vi "Example Solver.vi"(10 "Word List":string[](array[string])=["YELLOW", "ORANGE", "PURPLE", "BLUE", "GREEN", "RED"], 11 "Word Search Grid":string[][](array[string])=[["R", "B", "L", "U", "E", "W"], ["E", "G", "N", "A", "R", "O"], ["D", "B", "C", "E", "W", "L"], ["L", "L", "D", "K", "V", "L"], ["P", "U", "R", "P", "L", "E"], ["N", "E", "E", "R", "G", "Y"]]) -> (3 "Solutions":T1={"BLUE"=[{"Row"=0, "Column"=1}, {"Row"=0, "Column"=2}, {"Row"=0, "Column"=3}, {"Row"=0, "Column"=4}], "GREEN"=[{"Row"=5, "Column"=4}, {"Row"=5, "Column"=3}, {"Row"=5, "Column"=2}, {"Row"=5, "Column"=1}, {"Row"=5, "Column"=0}], "ORANGE"=[{"Row"=1, "Column"=5}, {"Row"=1, "Column"=4}, {"Row"=1, "Column"=3}, {"Row"=1, "Column"=2}, {"Row"=1, "Column"=1}, {"Row"=1, "Column"=0}], "PURPLE"=[{"Row"=4, "Column"=0}, {"Row"=4, "Column"=1}, {"Row"=4, "Column"=2}, {"Row"=4, "Column"=3}, {"Row"=4, "Column"=4}, {"Row"=4, "Column"=5}], "RED"=[{"Row"=0, "Column"=0}, {"Row"=1, "Column"=0}, {"Row"=2, "Column"=0}], "YELLOW"=[{"Row"=5, "Column"=5}, {"Row"=4, "Column"=5}, {"Row"=3, "Column"=5}, {"Row"=2, "Column"=5}, {"Row"=1, "Column"=5}, {"Row"=0, "Column"=5}]})   [LabVIEW 2023]
uses:
  Solutions--map.ctl
  Letter Index--cluster.ctl
panel:
  # "Do not change the connector pane of this VI."
  # "Observe the default values stored in this VI to understand how each word is represented in the Solutions map.\n\nSee the block diagram for a simple implementation of a solution. Note that this approach is not very efficient, and you will want to come up with a faster way to find the words in the grid."
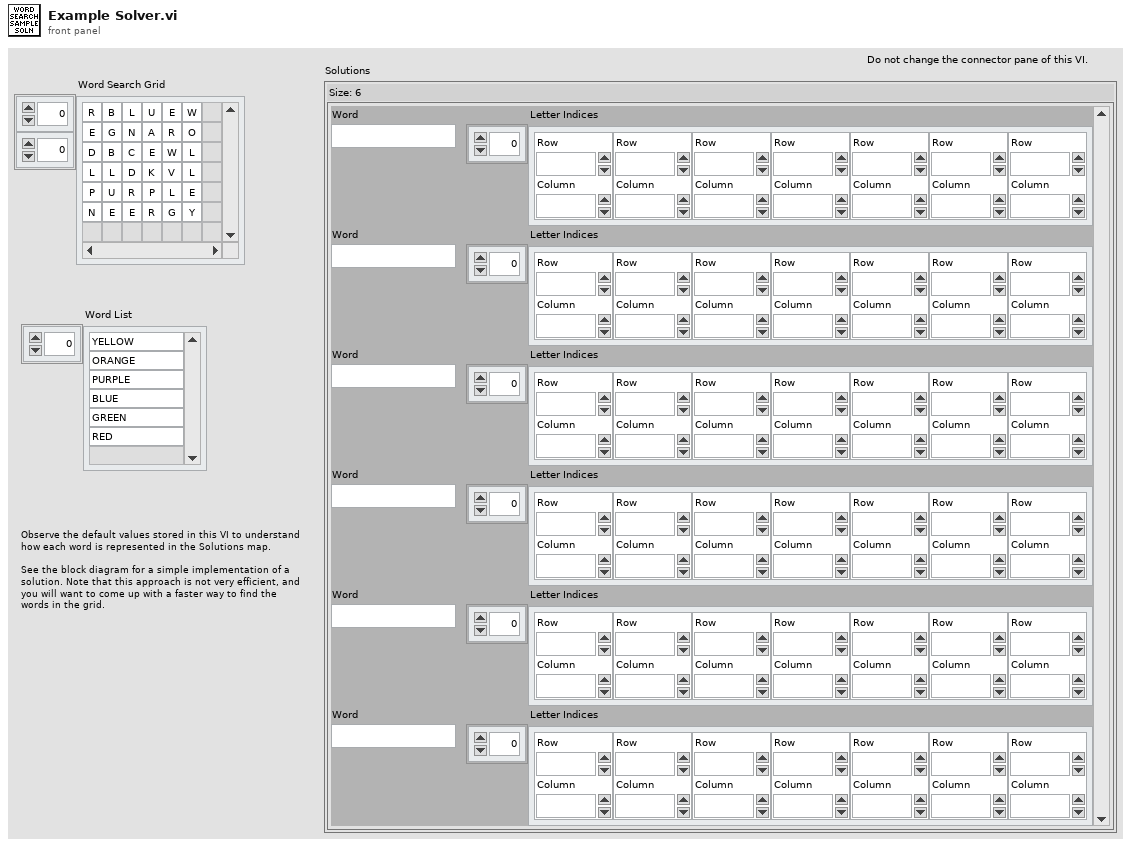
[diagram p1: front panel]
types:
  T1 = typedef "Solutions--map.ctl" = map{string, T2[]}
  T2 = typedef "Letter Index--cluster.ctl" = cluster{"Row":i32, "Column":i32}
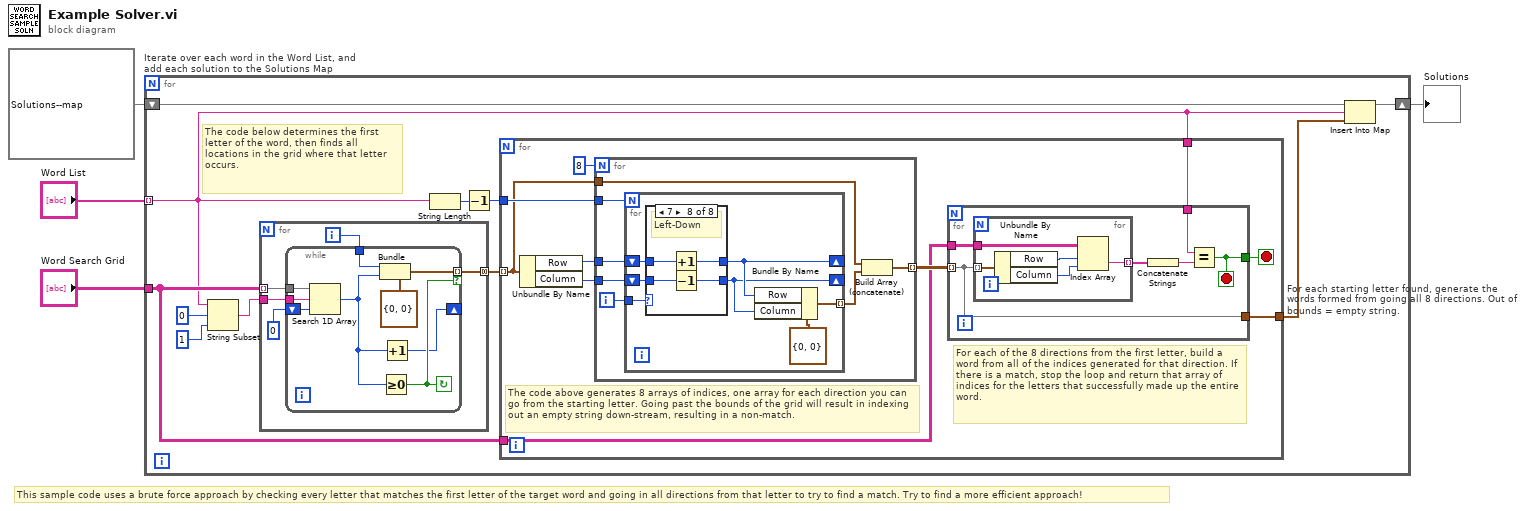
[diagram p0: block diagram]
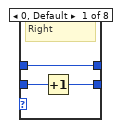
[diagram p2: hidden frame]
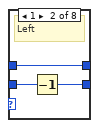
[diagram p3: hidden frame]
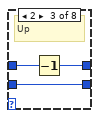
[diagram p4: hidden frame]
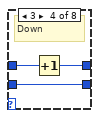
[diagram p5: hidden frame]
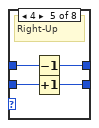
[diagram p6: hidden frame]
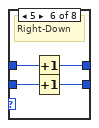
[diagram p7: hidden frame]
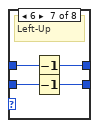
[diagram p8: hidden frame]
diagram:
  # "This sample code uses a brute force approach by checking every letter that matches the first letter of the target word and going in all directions from that letter to try to find a match. Try to find a more efficient approach!"
  n1 = for "Iterate over each word in the Word List, and add each solution to the Solutions Map" {
    tunnel: "Word Search Grid" -> [w7]
    tunnel: "Word List" -> [w6] mode=indexing
    shift-right: [w14] -> w4
    shift-left: T1 {} ("Solutions") -> [w15]
    # "The code below determines the first letter of the word, then finds all locations in the grid where that letter occurs."
    n2 = String Subset(string=w6, offset (0)=0, length (rest)=1 ("length (rest)")) -> (substring=w12:string)
    n3 = for {
      tunnel: w7 -> [w83] mode=indexing
      tunnel: w12 -> [w82]
      tunnel: [w80] -> w11 mode=concatenating
      i -> [w81]
      n4 = while {
        tunnel: w83 -> [w92]
        tunnel: w82 -> [w91]
        tunnel: w81 -> [w89]
        tunnel: [w88] -> w80 mode=indexing if=w87
        shift-right: [w84] -> _
        shift-left: 0 -> [w86]
        stop <- w87 continue-if-true
        n5 = Search 1D Array(1D array=w92, element=w91, start index (0)=w86) -> (index of element=w85:i32)
        n6 = Bundle(cluster=T2 {"Row"=0, "Column"=0} ("Letter Index"), "Row"=w89, "Column"=w85) -> (w88:T2)
        n7 = Greater Or Equal To 0?(x=w85) -> (x >= 0?=w87:bool)
        n8 = Increment(x=w85) -> (x+1=w84:i32)
      }
    }
    n9 = String Length(string=w6) -> (length=w9:i32)
    n10 = Decrement(x=w9) -> (x-1=w8:i32)
    n11 = for "For each starting letter found, generate the words formed from going all 8 directions. Out of bounds = empty string." {
      tunnel: w11 -> [w21] mode=indexing
      tunnel: w8 -> [w24]
      tunnel: w7 -> [w19]
      tunnel: [w18] -> w5
      tunnel: w6 -> [w17]
      stop <- w16 stop-if-true
      # "The code above generates 8 arrays of indices, one array for each direction you can go from the starting letter. Going past the bounds of the grid will result in indexing out an empty string down-stream, resulting in a non-match."
      # "For each of the 8 directions from the first letter, build a word from all of the indices generated for that direction. If there is a match, stop the loop and return that array of indices for the letters that successfully made up the entire word."
      n12 = Unbundle By Name(w21) -> ("Row"=w23:i32, "Column"=w22:i32)
      n13 = for {
        N: 8 -> [_]
        tunnel: w24 -> [w43]
        tunnel: w23 -> [w42]
        tunnel: w22 -> [w41]
        tunnel: w21 -> [w38]
        tunnel: [w37] -> w20 mode=indexing
        i -> [w40]
        n14 = for {
          N: w43 -> [_]
          tunnel: w40 -> [w48]
          tunnel: [w46] -> w39 mode=indexing
          shift-right: [w45] -> _
          shift-left: w42 -> [w50]
          shift-right: [w44] -> _
          shift-left: w41 -> [w49]
          n15 = case shown="7" w48 {
            tunnel: w50 -> [w51 w54 w58 w61 w65 w69 w73 w77]
            tunnel: w49 -> [w53 w56 w59 w62 w66 w70 w74 w78]
            tunnel: [w52 w55 w59 w62 w63 w67 w71 w75] -> w44
            tunnel: [w51 w54 w57 w60 w64 w68 w72 w76] -> w45
            frame 0, Default {
              # "Right"
              n16 = Increment(x=w53) -> (x+1=w52:i32)
            }
            frame 1 {
              # "Left"
              n17 = Decrement(x=w56) -> (x-1=w55:i32)
            }
            frame 2 {
              # "Up"
              n18 = Decrement(x=w58) -> (x-1=w57:i32)
            }
            frame 3 {
              # "Down"
              n19 = Increment(x=w61) -> (x+1=w60:i32)
            }
            frame 4 {
              # "Right-Up"
              n20 = Decrement(x=w65) -> (x-1=w64:i32)
              n21 = Increment(x=w66) -> (x+1=w63:i32)
            }
            frame 5 {
              # "Right-Down"
              n22 = Increment(x=w69) -> (x+1=w68:i32)
              n23 = Increment(x=w70) -> (x+1=w67:i32)
            }
            frame 6 {
              # "Left-Up"
              n24 = Decrement(x=w73) -> (x-1=w72:i32)
              n25 = Decrement(x=w74) -> (x-1=w71:i32)
            }
            frame 7 {
              # "Left-Down"
              n26 = Increment(x=w77) -> (x+1=w76:i32)
              n27 = Decrement(x=w78) -> (x-1=w75:i32)
            }
          }
          n28 = Bundle By Name(cluster=T2 {"Row"=0, "Column"=0} ("Letter Index"), "Row"=w45, "Column"=w44) -> (w46:T2)
        }
        n29 = Build Array (concatenate)(w38, w39) -> (w37:T2[])
      }
      n30 = for {
        tunnel: w20 -> [w28] mode=indexing
        tunnel: w19 -> [w31]
        tunnel: [w28] -> w18
        tunnel: w17 -> [w27]
        tunnel: [w26] -> w16
        stop <- w26 stop-if-true
        n31 = for {
          tunnel: w28 -> [w36] mode=indexing
          tunnel: w31 -> [w34]
          tunnel: [w32] -> w30 mode=indexing
          n32 = Unbundle By Name(w36) -> ("Row"=w35:i32, "Column"=w33:i32)
          n33 = Index Array(array=w34, index (row)=w35, index (col)=w33) -> (element=w32:string)
        }
        n34 = Concatenate Strings(w30) -> (w29:string)
        n35 = Equal?(x=w27, y=w29) -> (x = y?=w26:bool)
      }
    }
    n36 = Insert Into Map(map in=w15, key=w6, value=w5) -> (map out=w14:T1)  [unwired: 2 out]
  }
  "Solutions" <- w4
